vi "Lab Control Nov 2014.vi"() -> ()   [LabVIEW 2011]
uses:
  <vilib>/Utility/error.llb/DialogType.ctl
  <vilib>/DAQmx/write.llb/DAQmx Write (Analog 1D DBL 1Chan NSamp).vi
  <vilib>/DAQmx/write.llb/DAQmx Write (Digital 1D Wfm NChan NSamp).vi
  <vilib>/DAQmx/write.llb/DAQmx Write (Analog Wfm 1Chan NSamp).vi
  <vilib>/DAQmx/create/channels.llb/DAQmx Create Channel (DO-Digital Output).vi
  <vilib>/DAQmx/configure/timing.llb/DAQmx Timing (Sample Clock).vi
  <vilib>/DAQmx/configure/trigger.llb/DAQmx Start Trigger (Digital Edge).vi
  <vilib>/DAQmx/create/channels.llb/DAQmx Create Channel (CO-Pulse Generation-Time).vi
  <vilib>/DAQmx/create/channels.llb/DAQmx Create Channel (AO-Voltage-Basic).vi
  <vilib>/Waveform/WDTOps.llb/WDT Append Waveforms DBL.vi
  <vilib>/Waveform/DWDTOps.llb/DWDT Analog to Digital.vi
  <vilib>/Waveform/DWDTOps.llb/DWDT Append Digital Signals.vi
  <vilib>/DAQmx/miscellaneous.llb/DAQmx Fill In Error Info.vi
  <vilib>/Waveform/DWDTOps.llb/DWDT Uncompress Digital.vi
  <vilib>/measure/NI_MABase.lvlib
  Program Files (x86)/National Instruments/LabVIEW 2011/resource/objmgr/daqmx.rc
panel:
  out "Recording":bool=TRUE
  in  "Camera Trigger":bool=TRUE
  out "LASER":bool
  in  "Select Program":u16(ring) items=["Motor Control", "Wash Cycle"]
  in  "START/STOP\nMOTOR":bool=TRUE
  in  "RPM":dbl=180.0 min=0.0 max=1750.0 step=10.0
  out "Stop Duration":dbl=-10.0
  in  "START/STOP \nWASH CYCLE":bool=TRUE
  out "Stop Timer":i32=7
  in  "Go Duration":dbl=2.0
  in  "RPM":dbl=540.0 min=0.0 max=1750.0 step=10.0
  in  "Interval (min)":dbl=10.0
  out "Go Timer":i32=34
  in  "?":bool
  in  "VISA Output Motor Control":refnum<visa-resource-name>="COM1"
  in  "frequency":dbl=45.0 format="%0.2f"
  out "AO Mirror Signal (NOT IN REALTIME)":waveform(dbl)(graph)={"t0"=timestamp(0 s since 1904-01-01), "dt"=0.001, "Y"=array[1000 elements]}
  out "Camera Trigger":digitalwaveform(graph)={"t0"=timestamp(7.000000000000001 s since 1904-01-01), "dt"=2.2222222222222223e-05, "Y"={"transitions"=[0, 44999], "data"=[[0], [0]]}}
  out "Cutoff Signal":digitalwaveform(graph)={"t0"=timestamp(7.000000000000001 s since 1904-01-01), "dt"=2.2222222222222223e-05, "Y"={"transitions"=[0, 44999], "data"=[[0], [0]]}}
  in  "duty cycle (%)":dbl=100.0 format="%0.2f"
  in  "sampling info":cluster{"Fs":dbl, "#s":dbl}={"Fs"=45000.0, "#s"=45000.0} {"Fs" format="%.2p"}
  in  "phase":dbl format="%.2p"
  in  "amplitude":dbl=1.0 format="%0.2p"
  in  "frequency":dbl=45.0 format="%0.2p"
  in  "sampling info":cluster{"Fs":dbl, "#s":dbl}={"Fs"=45000.0, "#s"=45000.0} {"Fs" format="%.2p"}
  in  "phase":dbl=180.0 format="%.2p"
  in  "amplitude":dbl=1.0 format="%0.2p"
  in  "frequency":dbl=450.0 format="%0.2p"
  in  "sampling info":cluster{"Fs":dbl, "#s":dbl}={"Fs"=45000.0, "#s"=45000.0} {"Fs" format="%.2p"}
  in  "frequency":dbl=900.0 format="%0.2p"
  out "Actual AO Update Rate":dbl=45004.500450045 caption="Actual Update Generation Rate" format="%0.2f"
  in  "minimum value":dbl caption="Output Minimum Value" format="%0.2f"
  in  "maximum value":dbl=10.0 caption="Output Maximum Value" format="%0.2f"
  in  "physical channels":tag="Dev1/ao0" caption="Analog Output Mirror Control"
  out "DO Update Rate":dbl=45004.500450045 caption="Actual Input Rate" format="%0.2f"
  in  "Physical Channel":tag="Dev1/port0/line1" caption="Digital Output Laser Control"
  in  "Physical Channel 2":tag="Dev1/port0/line0" caption="Digital Output Camera Control"
  in  "DO Sample Clock Rate":dbl=45000.0 format="%0.2f"
  in  "stop":bool
  out "Camera & Laser Trigger":digitalwaveform(graph)={"t0"=timestamp(7.000000000000001 s since 1904-01-01), "dt"=2.2222222222222223e-05, "Y"={"transitions"=array[1801 elements], "data"=array1801x2[3602 elements]}}
  # "Select your output channels:\n1. Set Digital Output Laser Control to\n    Dev1/port0/line1\n2. Set Digital Output Camera Control to\n    Dev1/port0/line0\n3. Set Analog Output Mirror Control to\n    Dev1/ao0\n4. Set VISA Output Motor Control to\n    COM1\n5. Set the DO Sample Clock Rate\nIMPORTANT: USE THE SAME SAMPLING\nINFO FOR ALL DIGITAL OUTPUTS\n\nEMO (Emergency Off) terminates ALL\nsignals and stops the motor. Make sure\nto switch the laser to INT PRF SOURCE \nbefore or right after you hit EMO.\n\nThe laser gets triggered by this program \nas soon as you start it. When the green \nLASER-LED lights up, you can switch the\nlaser to EXT PRF SOURCE.\n\nThe Camera Trigger button starts or\nstops the camera trigger signal.\n\nIf you need to skip trigger signals, use\nthe Cutoff signal. Set the frequency to:\n           (camera frequency) / 10.\nYou can then use the phase and the \nduty cycle to adjust your signal (e.g.: \nwith a duty cycle of 80%, you skip every \nninth and tenth trigger signal).\n\nSelect which program you want to use:\n1. Motor Control:\n    Choose a value for RPM\n    180RPM = 3Hz in the motor\n                   = 1Hz in the tank\nHit the START/STOP MOTOR button\n2. Wash Cycle:\n    Again, choose RPM (for the wash\n    cycle)\n    - Interval (in minutes): Choose the\n      length of the interval\n    - Go Duration (in minutes): Sets how\n      long the motor is running during the\n      interval.\nAfter setting these values, hit\nSTART/STOP WASH CYCLE and the Go \nbutton.\nTo stop the motor, either hit the corres-\nponding START/STOP buttons or EMO"
  # "IO & Timing Options"
  # "Laser\nParameters"
  # "Camera\nParameters"
  # "Mirror\nParameters"
  # "Cutoff\nParameters"
  # "Motor\nParameters"
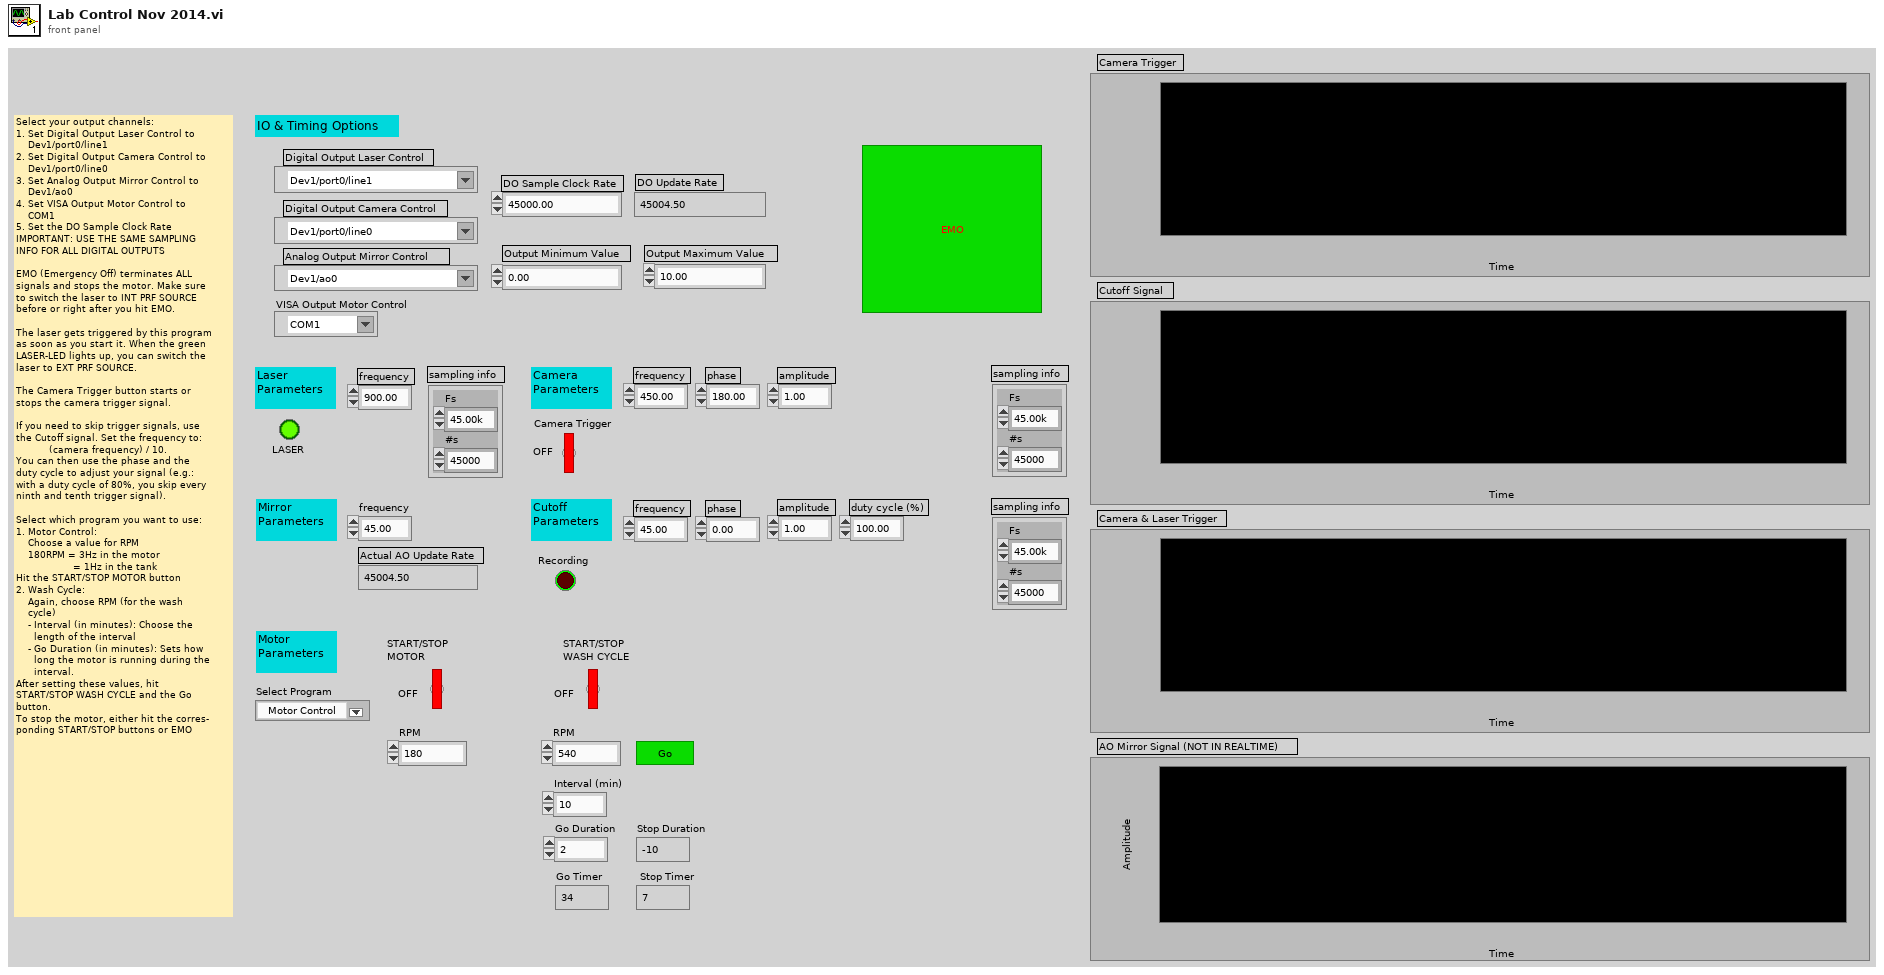
[diagram p1: front panel]
types:
  T1 = typedef "DialogType.ctl" = u16
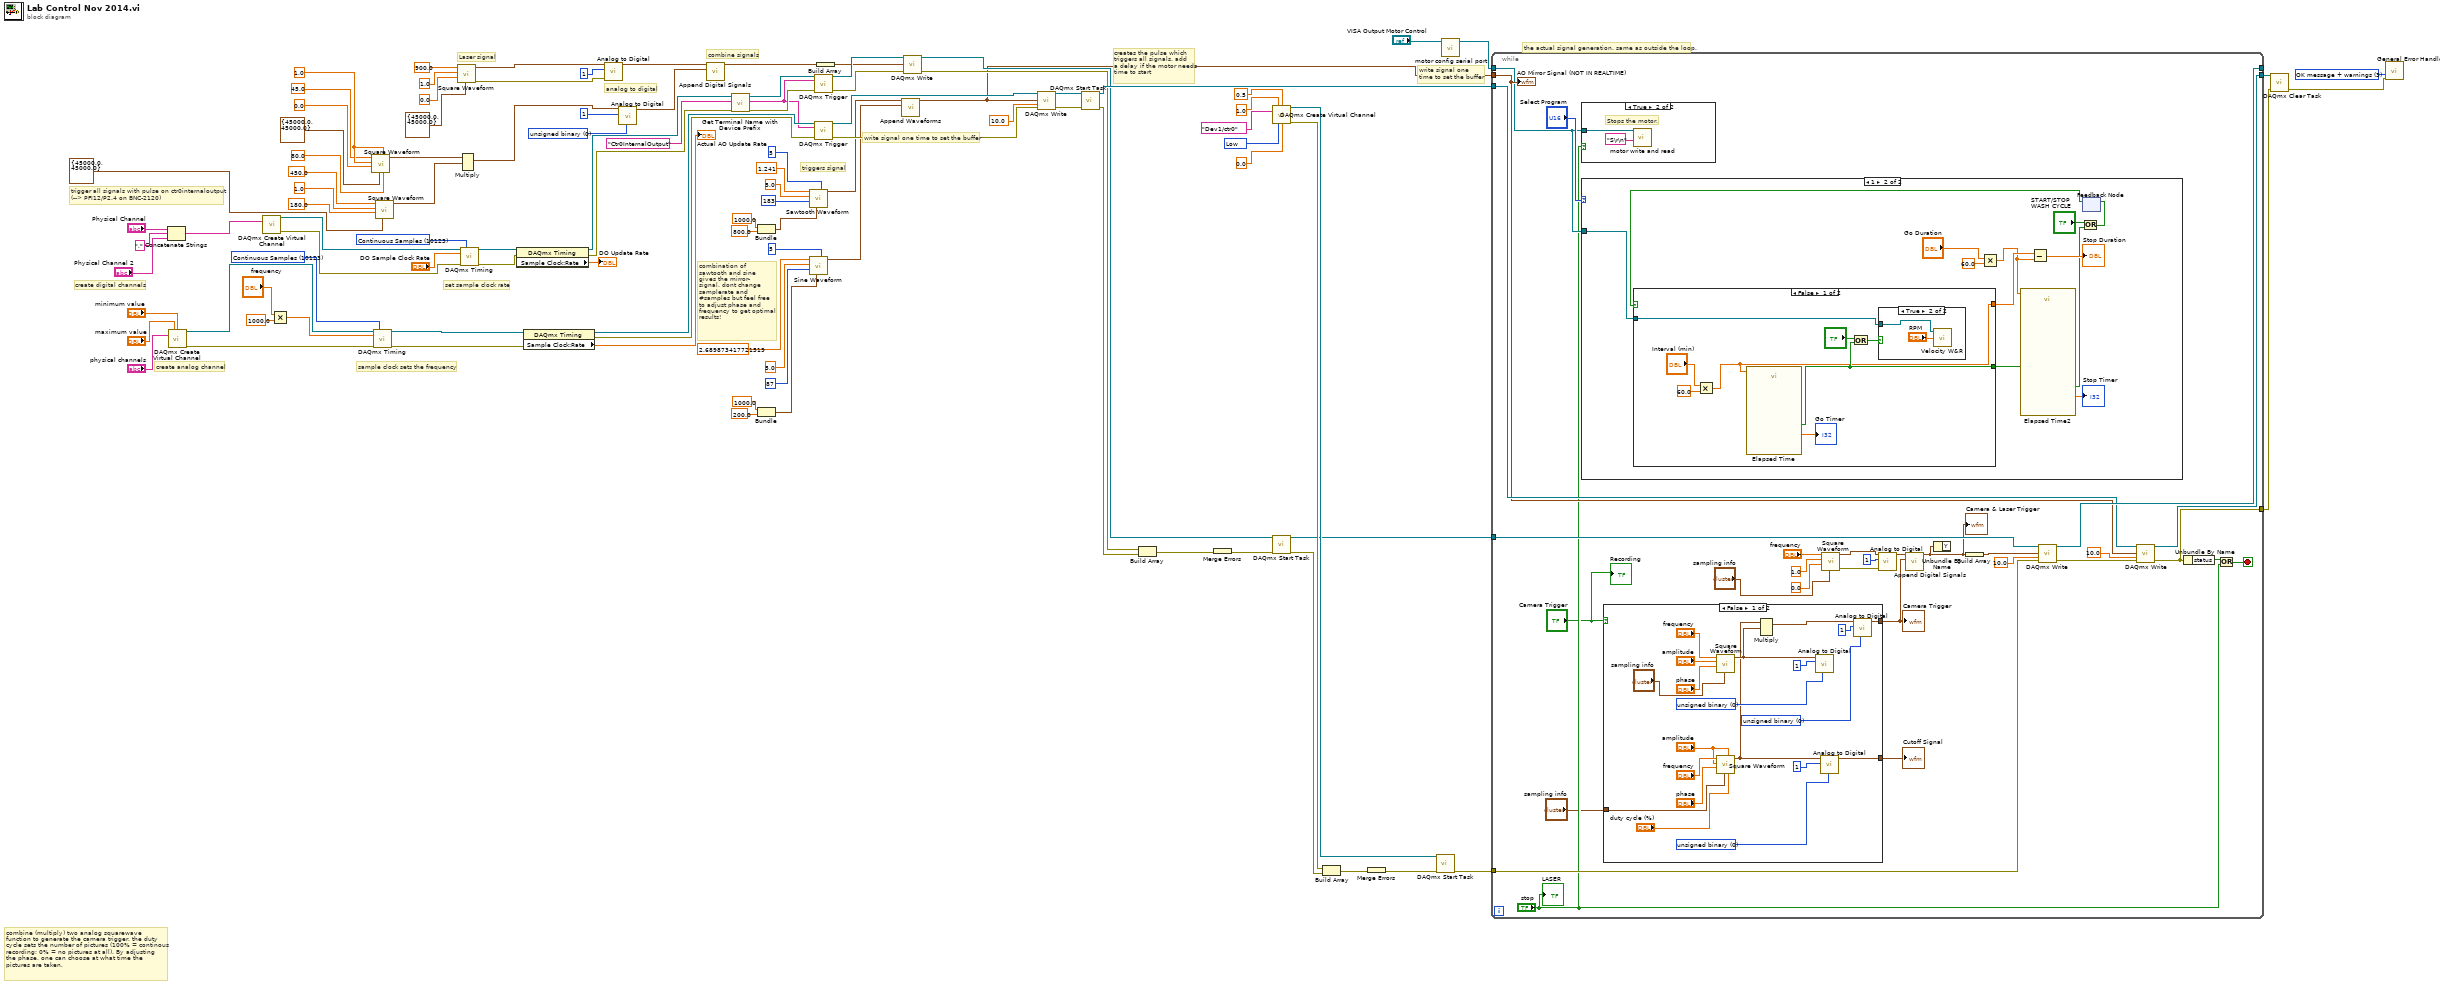
[diagram p0: block diagram]
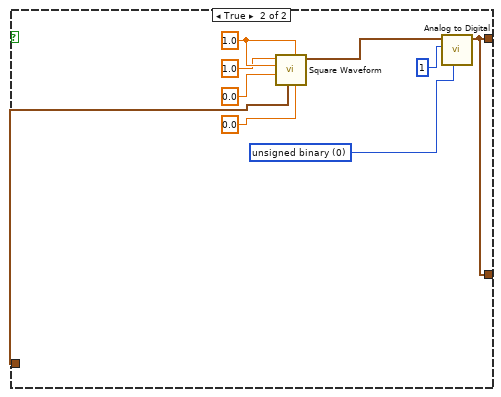
[diagram p2: hidden frame]
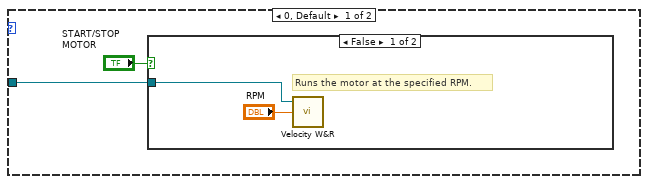
[diagram p4: hidden frame]
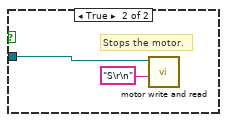
[diagram p5: hidden frame]
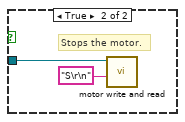
[diagram p7: hidden frame]
diagram:
  w53 = 1.0 ("amplitude")
  w28 = T1 3 items=["no dialog", "OK message", "continue or stop message", "OK message + warnings", "continue/stop + warnings"] ("type of dialog (OK msg:1)")
  w40 = u16 0 items=["unsigned binary", "offset binary", "2's complement"] ("data format (offset binary)")
  w54 = 10123 items=["Finite Samples"=10178, "Continuous Samples"=10123] ("sample mode")
  w84 = 10214 items=["High"=10192, "Low"=10214] ("Idle State")
  w97 = 10123 items=["Finite Samples"=10178, "Continuous Samples"=10123, "Hardware Timed Single Point"=12522] ("sample mode")
  # "the actual signal generation. same as outside the loop."
  # "creates the pulse which\ntriggers all signals. add\na delay if the motor needs\ntime to start"
  # "write signal one \ntime to set the buffer"
  # "write signal one time to set the buffer"
  # "triggers signal"
  # "combination of\nsawtooth and sine\ngives the mirror-\nsignal. dont change \nsamplerate and\n#samples but feel free\nto adjust phase and\nfrequency to get optimal\nresults!"
  # "sample clock sets the frequency"
  # "create analog channel"
  # "trigger all signals with pulse on ctr0internaloutput\n(--> PFI12/P2.4 on BNC-2120)"
  # "combine signals"
  # "analog to digital"
  # "Laser signal"
  # "combine (multiply) two analog squarewave \nfunction to generate the camera trigger. the duty \ncycle sets the number of pictures (100% = continous\nrecording; 0% = no pictures at all). By adjusting\nthe phase, one can choose at what time the\npictures are taken."
  # "set sample clock rate"
  # "create digital channels"
  n1 = Concatenate Strings("Physical Channel", ",", "Physical Channel 2") -> (w90:string)
  n2 = call-poly <vilib>:"DAQmx Create Virtual Channel.vi"("maximum value"="maximum value", "minimum value"="minimum value", "physical channels"="physical channels") -> ("task out"=w67:refnum<k21>, "error out"=w66:errorcluster)  [unwired: 6 in, 5 out]
  n3 = call-poly <vilib>:"DAQmx Create Virtual Channel.vi"("lines"=w90) -> ("task out"=w99:refnum<k21>, "error out"=w98:errorcluster)  [unwired: 13 in]
  n4 = Multiply(x="frequency", y=1000.0) -> (x*y=w1:dbl)
  n5 = call <vilib>:"Square Waveform.vi"("duty cycle (%)"=80.0, "offset"=w53, "sampling info"=cluster{"Fs":dbl, "#s":dbl} {"Fs"=45000.0, "#s"=45000.0}, "phase"=0.0, "amplitude"=w53, "frequency"=45.0) -> ("signal out"=w52:waveform(dbl))  [unwired: 4 in, 1 out]
  n6 = call-poly <vilib>:"DAQmx Timing.vi"("task/channels in"=w67, "sample mode"=w54, "rate"=w1, "error in"=w66) -> ("task out"=w62:refnum<k21>, "error out"=w61:errorcluster)  [unwired: 3 in, 7 out]
  n7 = call <vilib>:"Square Waveform.vi"("sampling info"=cluster{"Fs":dbl, "#s":dbl} {"Fs"=45000.0, "#s"=45000.0}, "phase"=180.0, "amplitude"=1.0, "frequency"=450.0) -> ("signal out"=w49:waveform(dbl))  [unwired: 6 in, 1 out]
  n8 = call <vilib>:"Square Waveform.vi"("sampling info"=cluster{"Fs":dbl, "#s":dbl} {"Fs"=45000.0, "#s"=45000.0}, "phase"=0.0, "amplitude"=1.0, "frequency"=900.0) -> ("error out"=w103:errorcluster, "signal out"=w104:waveform(dbl))  [unwired: 6 in]
  n9 = Multiply(1:w49, 2:w52) -> (0:w51:waveform(dbl))  [unwired: 1 in, 1 out]
  n10 = call-poly <vilib>:"DAQmx Timing.vi"("task/channels in"=w99, "sample mode"=w97, "rate"="DO Sample Clock Rate", "error in"=w98) -> ("task out"=w8:refnum<k21>, "error out"=w6:errorcluster)  [unwired: 10 in]
  n11 = property class="DAQmx Timing"(reference=w8, error in=w6) -> (reference out=w7:refnum<k21>, error out=w5:errorcluster, "Sample Clock:Rate"=→"DO Update Rate":dbl)
  n12 = property class="DAQmx Timing"(reference=w62, error in=w61) -> (reference out=w59:refnum<k21>, error out=w57:errorcluster, "Sample Clock:Rate"=→"Actual AO Update Rate":dbl)
  n13 = call-poly <vilib>:"Analog to Digital.vi"("error in (no error)"=w103, "resolution (16 bit)"=1, "analog waveform"=w104) -> ("digital waveform"=w38:digitalwaveform)  [unwired: 5 in, 3 out]
  n14 = call-poly <vilib>:"Analog to Digital.vi"("data format (offset binary)"=w40, "resolution (16 bit)"=1, "analog waveform"=w51) -> ("digital waveform"=w39:digitalwaveform)  [unwired: 5 in, 3 out]
  n15 = call-poly <vilib>:"Append Digital Signals.vi"("digital waveform (low bits)"=w39, "digital waveform (high bits)"=w38) -> ("digital waveform out"=w37:digitalwaveform)  [unwired: 8 in, 1 out]
  n16 = call "Get Terminal Name with Device Prefix.vi"("error in (no error)"=w5, "Local Terminal Name"="Ctr0InternalOutput" ("terminal"), "task/channels in"=w7) -> ("error out"=w87:errorcluster, "Terminal Name with Device Prefix"=w35:tag, "task out"=w88:refnum<k21>)  [unwired: 1 in, 5 out]
  n17 = Bundle("x"=1000.0, "x"=800.0) -> (w14:cluster{"x":dbl, "x":dbl})  [unwired: 1 in]
  n18 = Bundle("x"=1000.0, "x"=200.0) -> (w11:cluster{"x":dbl, "x":dbl})  [unwired: 1 in]
  n19 = call <vilib>:"Sawtooth Waveform.vi"("offset"=5, "sampling info"=w14, "phase"=183 ("Sawtooth Phase"), "amplitude"=5.0 ("sawtooth amp"), "frequency"=1.241 ("Sawtooth Frequency")) -> ("signal out"=w19:waveform(dbl))  [unwired: 5 in, 1 out]
  n20 = call <vilib>:"Sine Waveform.vi"("offset"=5, "sampling info"=w11, "phase"=87 ("Sin Phase"), "amplitude"=5.0 ("sin amp"), "frequency"=2.689873417721519 ("Sin Frequency")) -> ("signal out"=w18:waveform(dbl))  [unwired: 5 in, 1 out]
  n21 = call-poly <vilib>:"DAQmx Trigger.vi"("task/channels in"=w88, "source"=w35, "error in"=w87) -> ("task out"=w86:refnum<k21>, "error out"=w85:errorcluster)  [unwired: 2 in, 9 out]
  n22 = call-poly <vilib>:"DAQmx Trigger.vi"("task/channels in"=w59, "source"=w35, "error in"=w57) -> ("task out"=w58:refnum<k21>, "error out"=w56:errorcluster)  [unwired: 2 in, 9 out]
  n23 = Build Array(w37) -> (w36:digitalwaveform[])
  n24 = call-poly <vilib>:"Append Waveforms.vi"("waveform B"=w18, "waveform A"=w19) -> ("waveform out"=w17:waveform(dbl))  [unwired: 8 in, 1 out]
  n25 = call-poly <vilib>:"DAQmx Write.vi"("task/channels in"=w86, "data"=w36, "error in"=w85) -> ("task out"=w33:refnum<k21>, "error out"=w32:errorcluster)  [unwired: 10 in, 1 out]
  n26 = call-poly <vilib>:"DAQmx Write.vi"("task/channels in"=w58, "data"=w17, "timeout"=10.0 ("Wirite Timeout"), "error in"=w56) -> ("task out"=w64:refnum<k21>, "error out"=w63:errorcluster)  [unwired: 1 in, 9 out]
  n27 = call <vilib>:"DAQmx Start Task.vi"("task/channels in"=w64, "error in"=w63) -> ("task out"=w34:refnum<k21>, "error out"=w55:errorcluster)  [unwired: 12 out]
  n28 = Build Array(w32, w55) -> (w75:errorcluster[])
  n29 = Merge Errors(w75) -> (w76:errorcluster)
  n30 = call-poly <vilib>:"DAQmx Create Virtual Channel.vi"("high time"=1.0 ("High Time"), "low time"=0.5 ("Low Time"), "counter"=tag "Dev1/ctr0" ("Counter(s)"), "idle state"=w84, "initial delay"=0.0 ("Initial Delay")) -> ("task out"=w73:refnum<k21>, "error out"=w79:errorcluster)  [unwired: 4 in, 5 out]
  n31 = call <vilib>:"DAQmx Start Task.vi"("task/channels in"=w33, "error in"=w76) -> ("task out"=w72:refnum<k21>, "error out"=w74:errorcluster)  [unwired: 12 out]
  n32 = Build Array(w79, w74) -> (w78:errorcluster[])
  n33 = Merge Errors(w78) -> (w77:errorcluster)
  n34 = call <vilib>:"DAQmx Start Task.vi"("task/channels in"=w73, "error in"=w77) -> ("error out"=w71:errorcluster)  [unwired: 13 out]
  n35 = call "motor config serial port.vi"("VISA resource name in"="VISA Output Motor Control") -> ("VISA resource name out"=w9:refnum<visa-resource-name>)  [unwired: 9 in, 1 out]
  n36 = while {
    tunnel: w72 -> [w132]
    tunnel: [w129] -> _
    tunnel: w71 -> [w131]
    tunnel: [w125] -> w30
    tunnel: w34 -> [w128]
    tunnel: [w124] -> w31
    tunnel: w17 -> [w120]
    tunnel: w9 -> [w118]
    stop <- w123 stop-if-true
    n37 = case shown="True" "stop" {
      tunnel: w118 -> [_ w163]
      frame False {
      }
      frame True {
        # "Stops the motor."
        n38 = call "motor write and read.vi"("VISA resource name in"=w163, "Write String"="S\r\n") -> ()  [unwired: 2 in, 5 out]
      }
    }
    n39 = case shown="1" "Select Program" {
      tunnel: w118 -> [w165 w174]
      frame 0, Default {
        n40 = case shown="False" "START/STOP\nMOTOR" {
          tunnel: w165 -> [w168 w169]
          frame False {
            # "Runs the motor at the specified RPM."
            n41 = call "Velocity W&R.vi"("RPM"="RPM", "VISA resource name in"=w168) -> ()  [unwired: 1 in, 2 out]
          }
          frame True {
            # "Stops the motor."
            n42 = call "motor write and read.vi"("VISA resource name in"=w169, "Write String"="S\r\n") -> ()  [unwired: 2 in, 5 out]
          }
        }
      }
      frame 1 {
        n43 = Multiply(x="Go Duration", y=60.0) -> (x*y=w171:dbl)
        n44 = feedback #1() -> (w180:bool)  [unwired: 1 in]
        n45 = case shown="False" w180 {
          tunnel: w174 -> [w190 w193]
          tunnel: [w187 _] -> w176
          tunnel: [w183 _] -> w182
          frame False {
            n46 = Multiply(x="Interval (min)", y=60.0) -> (x*y=w183:dbl)
            n47 = call "Elapsed Time"("Time Target (s)"=w183) -> ("Elapsed Time (s)"=→"Go Timer":dbl, "Time has Elapsed"=w187:bool)  [unwired: 11 in, 6 out]
            n48 = Or(x="?", y=w187) -> (x .or. y?=w186:bool)
            n49 = case shown="True" w186 {
              tunnel: w190 -> [_ w192]
              frame False {
              }
              frame True {
                n50 = call "Velocity W&R.vi"("RPM"="RPM", "VISA resource name in"=w192) -> ()  [unwired: 1 in, 2 out]
              }
            }
          }
          frame True {
            # "Stops the motor."
            n51 = call "motor write and read.vi"("VISA resource name in"=w193, "Write String"="S\r\n") -> ()  [unwired: 2 in, 5 out]
          }
        }
        n52 = call "Elapsed Time2"("Time Target (s)"=w171, "Reset"=w176) -> ("Elapsed Time (s)"=→"Stop Timer":dbl, "Time has Elapsed"=w177:bool)  [unwired: 10 in, 6 out]
        n53 = Subtract(x=w182, y=w171) -> (x-y=→"Stop Duration":dbl)
        n54 = Or(x="START/STOP \nWASH CYCLE", y=w177) -> (x .or. y?=w179:bool)
        n55 = feedback-in #1(w179) -> ()
      }
    }
    n56 = case shown="False" "Camera Trigger" {
      tunnel: [w136 w154] -> w108
      tunnel: [w135 w154] -> w107
      tunnel: "sampling info" -> [w134 w155]
      frame False {
        w150 = u16 0 items=["unsigned binary", "offset binary", "2's complement"] ("data format (offset binary)")
        w149 = u16 0 items=["unsigned binary", "offset binary", "2's complement"] ("data format (offset binary)")
        w146 = u16 0 items=["unsigned binary", "offset binary", "2's complement"] ("data format (offset binary)")
        n57 = call <vilib>:"Square Waveform.vi"("sampling info"="sampling info", "phase"="phase", "amplitude"="amplitude", "frequency"="frequency") -> ("signal out"=w148:waveform(dbl))  [unwired: 6 in, 1 out]
        n58 = call <vilib>:"Square Waveform.vi"("duty cycle (%)"="duty cycle (%)", "offset"="amplitude", "sampling info"=w134, "phase"="phase", "amplitude"="amplitude", "frequency"="frequency") -> ("signal out"=w147:waveform(dbl))  [unwired: 4 in, 1 out]
        n59 = Multiply(1:w148, 2:w147) -> (0:w138:waveform(dbl))  [unwired: 1 in, 1 out]
        n60 = call-poly <vilib>:"Analog to Digital.vi"("data format (offset binary)"=w150, "resolution (16 bit)"=1, "analog waveform"=w148) -> ()  [unwired: 5 in, 4 out]
        n61 = call-poly <vilib>:"Analog to Digital.vi"("data format (offset binary)"=w149, "resolution (16 bit)"=1, "analog waveform"=w147) -> ("digital waveform"=w136:digitalwaveform)  [unwired: 5 in, 3 out]
        n62 = call-poly <vilib>:"Analog to Digital.vi"("data format (offset binary)"=w146, "resolution (16 bit)"=1, "analog waveform"=w138) -> ("digital waveform"=w135:digitalwaveform)  [unwired: 5 in, 3 out]
      }
      frame True {
        w162 = 1.0 ("amplitude 2")
        w158 = u16 0 items=["unsigned binary", "offset binary", "2's complement"] ("data format (offset binary)")
        n63 = call <vilib>:"Square Waveform.vi"("duty cycle (%)"=0.0 ("duty cycle (%) 2"), "offset"=w162, "sampling info"=w155, "phase"=0.0 ("phase 2"), "amplitude"=w162, "frequency"=1.0 ("frequency 2")) -> ("signal out"=w159:waveform(dbl))  [unwired: 4 in, 1 out]
        n64 = call-poly <vilib>:"Analog to Digital.vi"("data format (offset binary)"=w158, "resolution (16 bit)"=1, "analog waveform"=w159) -> ("digital waveform"=w154:digitalwaveform)  [unwired: 5 in, 3 out]
      }
    }
    "Cutoff Signal" <- w108
    "Camera Trigger" <- w107
    n65 = call <vilib>:"Square Waveform.vi"("sampling info"="sampling info", "phase"=0.0, "amplitude"=1.0, "frequency"="frequency") -> ("error out"=w115:errorcluster, "signal out"=w116:waveform(dbl))  [unwired: 6 in]
    n66 = call-poly <vilib>:"Analog to Digital.vi"("error in (no error)"=w115, "resolution (16 bit)"=1, "analog waveform"=w116) -> ("digital waveform"=w109:digitalwaveform)  [unwired: 5 in, 3 out]
    n67 = call-poly <vilib>:"Append Digital Signals.vi"("digital waveform (low bits)"=w107, "digital waveform (high bits)"=w109) -> ("digital waveform out"=w121:digitalwaveform)  [unwired: 8 in, 1 out]
    "Camera & Laser Trigger" <- w121
    n68 = Unbundle By Name(w121) -> ()  [unwired: 1 out]
    n69 = Build Array(w121) -> (w122:digitalwaveform[])
    n70 = call-poly <vilib>:"DAQmx Write.vi"("task/channels in"=w132, "data"=w122, "timeout"=10.0, "error in"=w131) -> ("task out"=w129:refnum<k21>, "error out"=w126:errorcluster)  [unwired: 9 in, 1 out]
    n71 = call-poly <vilib>:"DAQmx Write.vi"("task/channels in"=w128, "data"=w120, "timeout"=10.0, "error in"=w126) -> ("task out"=w124:refnum<k21>, "error out"=w125:errorcluster)  [unwired: 9 in, 1 out]
    n72 = Unbundle By Name(w125) -> ("status"=w133:bool)
    n73 = Or(x=w133, y="stop") -> (x .or. y?=w123:bool)
    "AO Mirror Signal (NOT IN REALTIME)" <- w120
    "LASER" <- "stop"
    "Recording" <- "Camera Trigger"
  }
  n74 = call <vilib>:"DAQmx Clear Task.vi"("task in"=w31, "error in"=w30) -> ("error out"=w29:errorcluster)  [unwired: 13 in]
  n75 = call <vilib>:"General Error Handler.vi"("type of dialog (OK msg:1)"=w28, "error in (no error)"=w29) -> ()  [unwired: 14 out]
